vi "Unrock_Data_To_Cluster.vi"(0 "Test":sgl[][](array[numeric]), 1 "Dev":sgl[](array[numeric]), 2 "Inacc":sgl[](array[numeric]), 3 "DIN":string, 4 "HN":string[](array[string]), 5 "HS":sgl[](array[numeric]), 6 "TEMP":string, 7 "TV":sgl[][](array[numeric]), 8 "TSN":string, 9 "HV":sgl[](array[numeric]), 10 "MODE":string, 11 "REP":sgl[](array[numeric]), 13 "AVG":sgl[](array[numeric])) -> (14 "All_data_String":string[][](array[string]), 15 "输出簇":T1)   [LabVIEW 2019]
uses:
  Unrock_Cluster.ctl
  Test_load.ctl
  Hardness_test.ctl
  TEST.lvclass
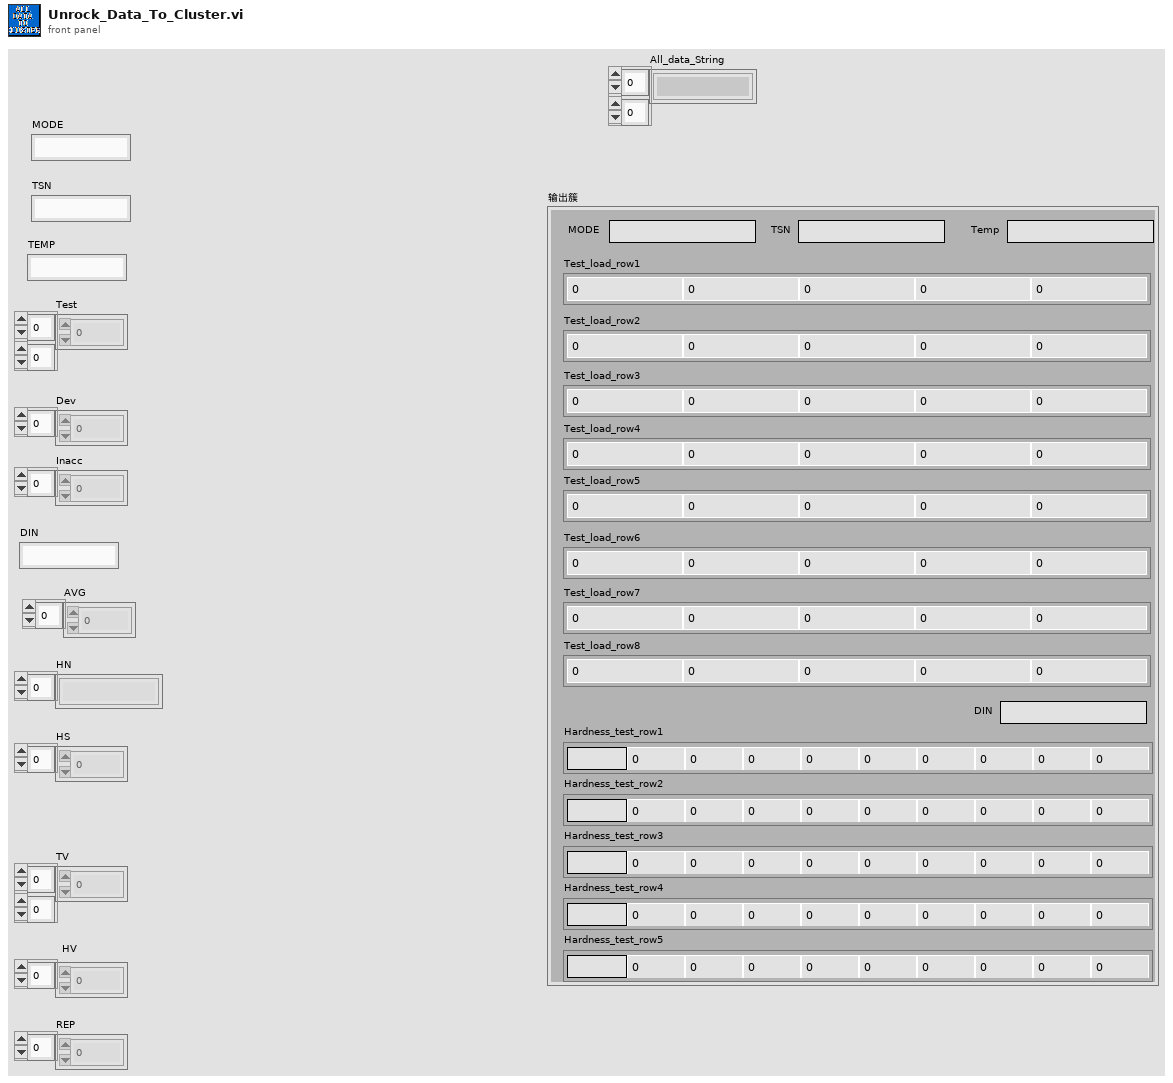
[diagram p1: front panel]
types:
  T1 = typedef "TEST.lvclass/Unrock_Cluster.ctl" = cluster{"MODE":string, "TSN":string, "Temp":string, "Test_load_row1":T2, "Test_load_row2":T2, "Test_load_row3":T2, "Test_load_row4":T2, "Test_load_row5":T2, "Test_load_row6":T2, "Test_load_row7":T2, "Test_load_row8":T2, "DIN":string, "Hardness_test_row1":T3, "Hardness_test_row2":T3, "Hardness_test_row3":T3, "Hardness_test_row4":T3, "Hardness_test_row5":T3}
  T2 = typedef "TEST.lvclass/Test_load.ctl" = cluster{"TEST1":sgl, "TEST2":sgl, "TEST3":sgl, "DEV":sgl, "INACC":sgl}
  T3 = typedef "TEST.lvclass/Hardness_test.ctl" = cluster{"HN":string, "HS":sgl, "TV1":sgl, "TV2":sgl, "TV3":sgl, "TV4":sgl, "TV5":sgl, "AVG":sgl, "HV":sgl, "REP":sgl}
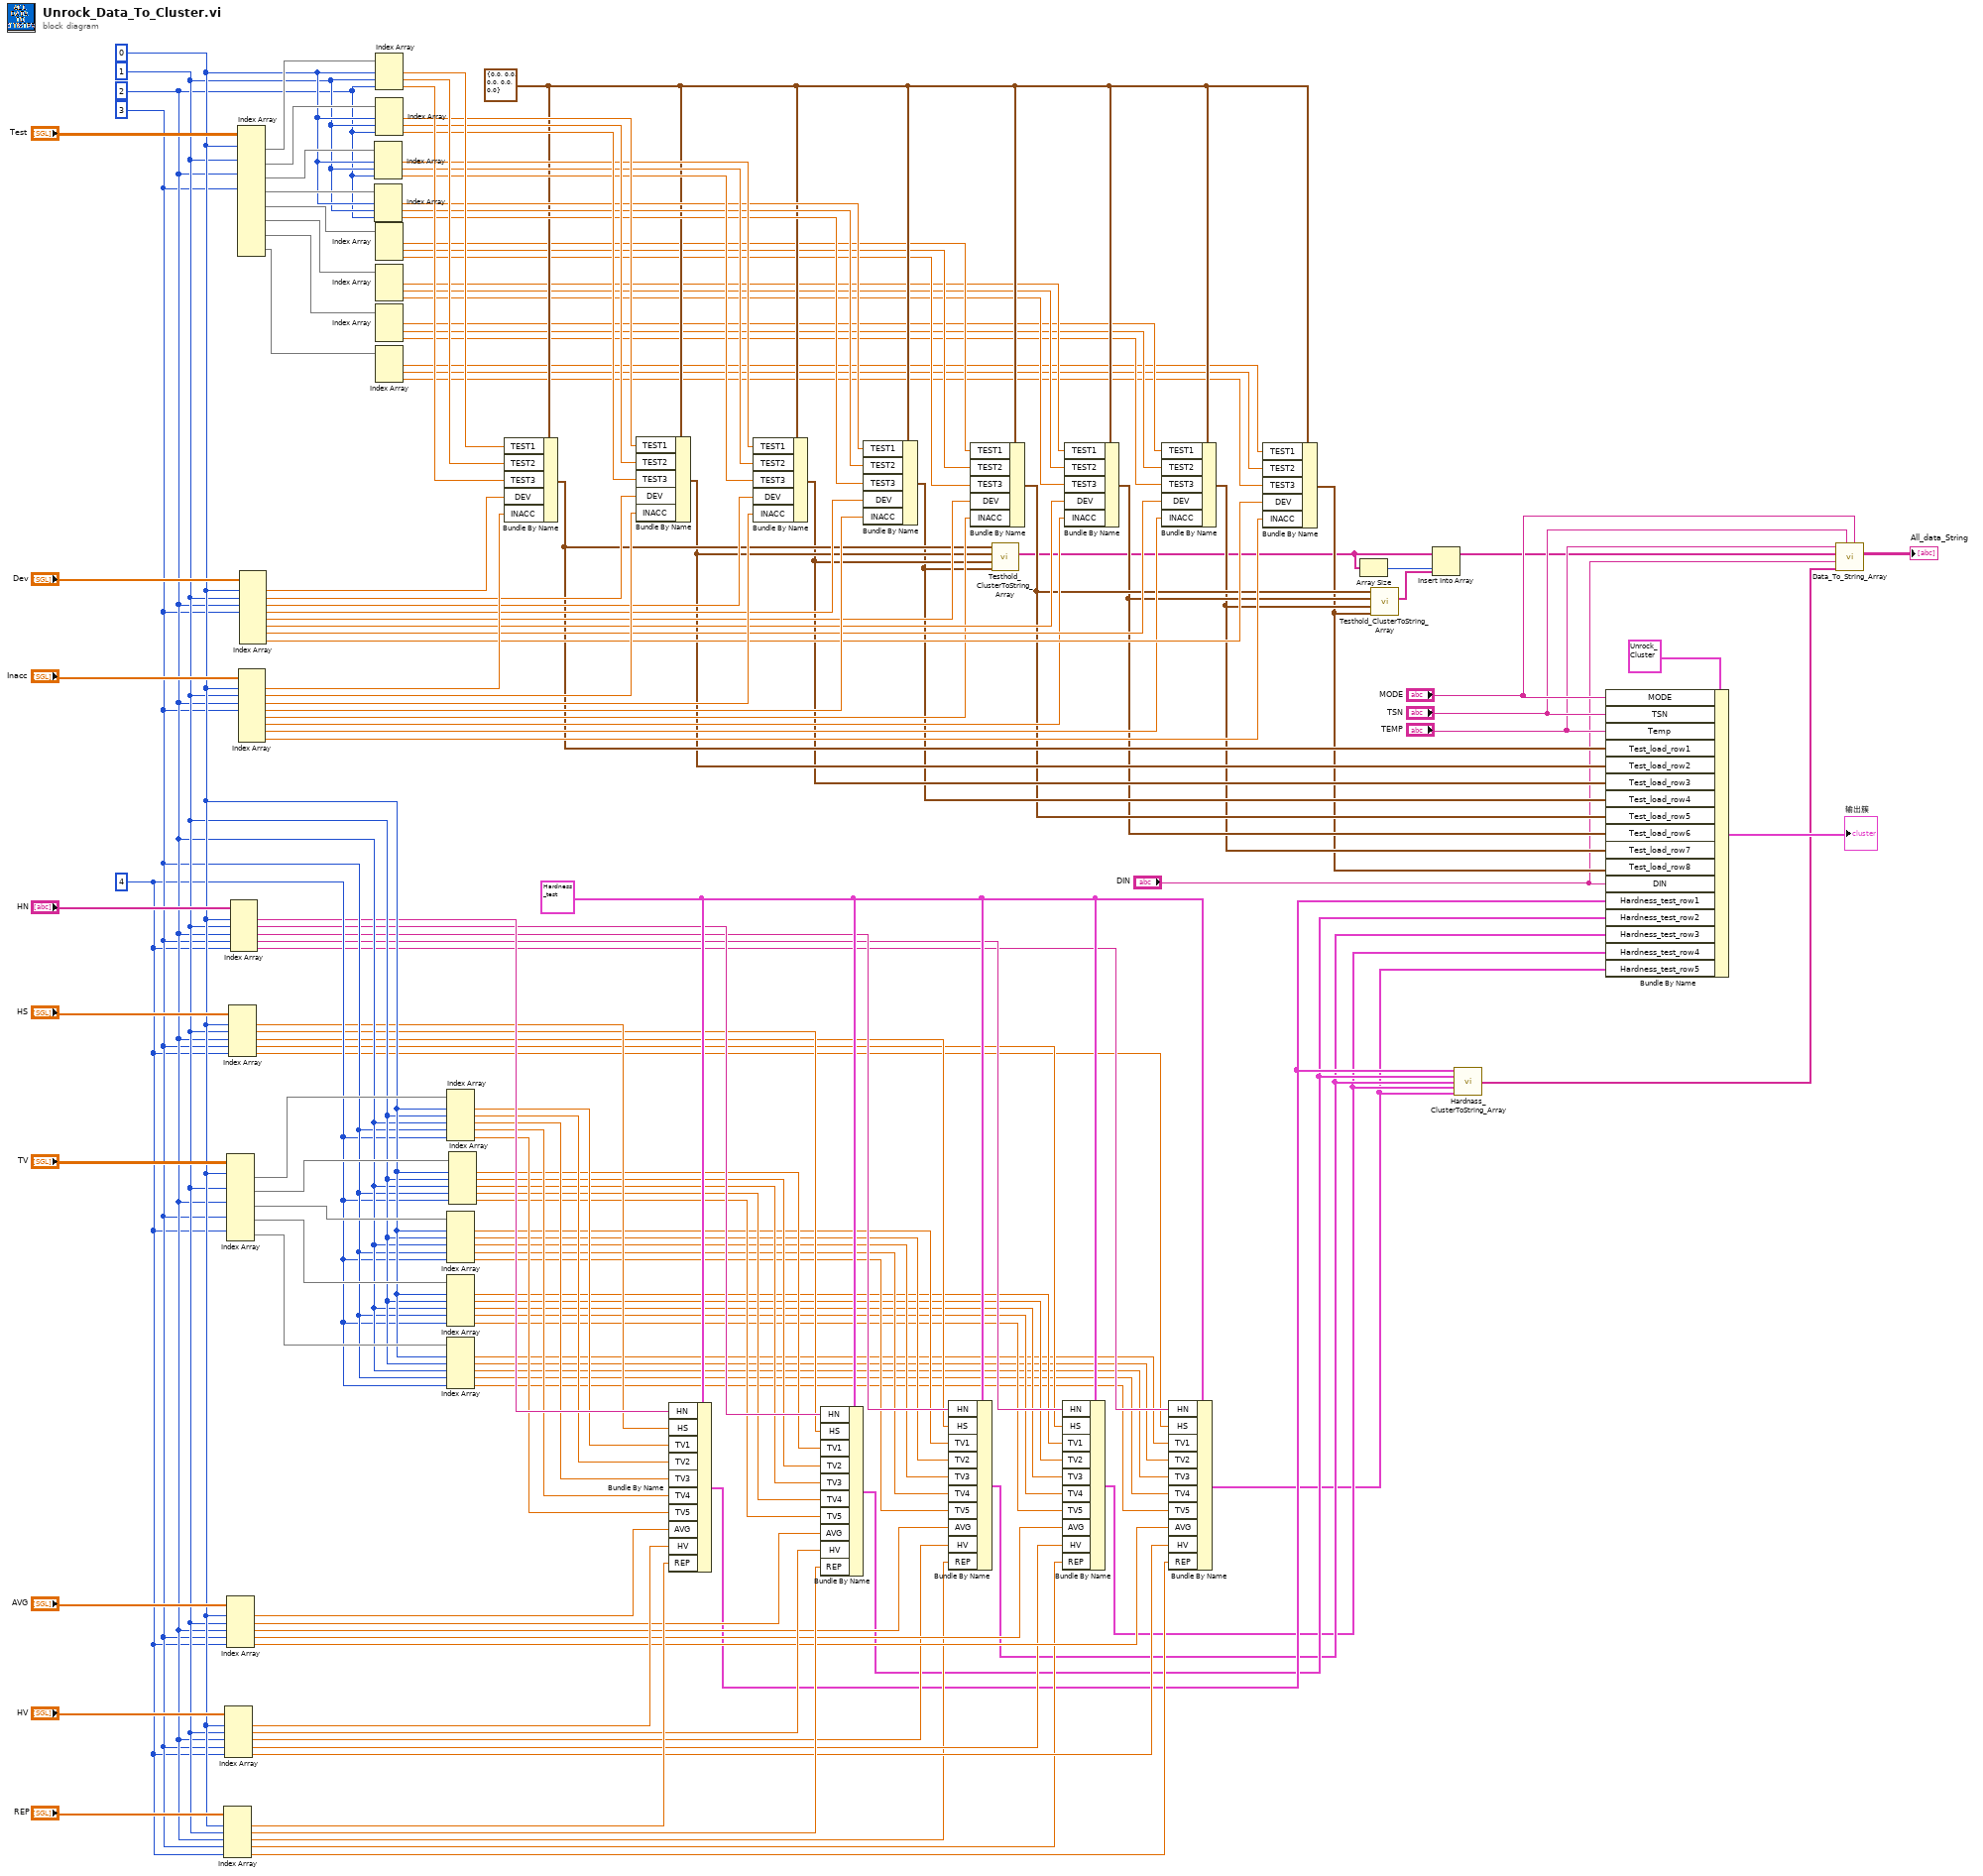
[diagram p0: block diagram]
diagram:
  w96 = T3 {"HN"="", "HS"=0.0, "TV1"=0.0, "TV2"=0.0, "TV3"=0.0, "TV4"=0.0, "TV5"=0.0, "AVG"=0.0, "HV"=0.0, "REP"=0.0} ("Hardness_test")
  w102 = 4
  w43 = T2 {"TEST1"=0.0, "TEST2"=0.0, "TEST3"=0.0, "DEV"=0.0, "INACC"=0.0} ("Test_load")
  w103 = 3 ("索引 (行)")
  w104 = 2 ("索引 (行)")
  w105 = 1 ("索引 (行)")
  w106 = 0 ("索引 (行)")
  n1 = Index Array(array="REP", index #1=w106, index #2=w105, index #3=w104, index #4=w103, index #5=w102) -> (element #1=w97:sgl, element #2=w91:sgl, element #3=w78:sgl, element #4=w77:sgl, element #5=w76:sgl)
  n2 = Index Array(array="HV", index #1=w106, index #2=w105, index #3=w104, index #4=w103, index #5=w102) -> (element #1=w98:sgl, element #2=w92:sgl, element #3=w81:sgl, element #4=w80:sgl, element #5=w79:sgl)
  n3 = Index Array(array="TV", index (row) #1=w106, index (row) #2=w105, index (row) #3=w104, index (row) #4=w103, index (row) #5=w102) -> (element #1=w111:sgl[], element #2=w110:sgl[], element #3=w109:sgl[], element #4=w108:sgl[], element #5=w107:sgl[])  [unwired: 5 in]
  n4 = Index Array(array="AVG", index #1=w106, index #2=w105, index #3=w104, index #4=w103, index #5=w102) -> (element #1=w99:sgl, element #2=w93:sgl, element #3=w84:sgl, element #4=w83:sgl, element #5=w82:sgl)
  n5 = Index Array(array="HS", index #1=w106, index #2=w105, index #3=w104, index #4=w103, index #5=w102) -> (element #1=w100:sgl, element #2=w94:sgl, element #3=w87:sgl, element #4=w86:sgl, element #5=w85:sgl)
  n6 = Index Array(array="HN", index #1=w106, index #2=w105, index #3=w104, index #4=w103, index #5=w102) -> (element #1=w101:string, element #2=w95:string, element #3=w90:string, element #4=w89:string, element #5=w88:string)
  n7 = Index Array(array="Test", index (row) #1=w106, index (row) #2=w105, index (row) #3=w104, index (row) #4=w103) -> (element #1=w141:sgl[], element #2=w140:sgl[], element #3=w139:sgl[], element #4=w138:sgl[], element #5=w42:sgl[], element #6=w41:sgl[], element #7=w40:sgl[], element #8=w39:sgl[])  [unwired: 12 in]
  n8 = Index Array(array="Inacc", index #1=w106, index #2=w105, index #3=w104, index #4=w103) -> (element #1=w133:sgl, element #2=w122:sgl, element #3=w120:sgl, element #4=w118:sgl, element #5=w22:sgl, element #6=w21:sgl, element #7=w20:sgl, element #8=w19:sgl)  [unwired: 4 in]
  n9 = Index Array(array="Dev", index #1=w106, index #2=w105, index #3=w104, index #4=w103) -> (element #1=w134:sgl, element #2=w123:sgl, element #3=w121:sgl, element #4=w119:sgl, element #5=w26:sgl, element #6=w25:sgl, element #7=w24:sgl, element #8=w23:sgl)  [unwired: 4 in]
  n10 = Index Array(array=w139, index #1=w106, index #2=w105, index #3=w104) -> (element #1=w129:sgl, element #2=w128:sgl, element #3=w127:sgl)
  n11 = Index Array(array=w138, index #1=w106, index #2=w105, index #3=w104) -> (element #1=w126:sgl, element #2=w125:sgl, element #3=w124:sgl)
  n12 = Index Array(array=w141, index #1=w106, index #2=w105, index #3=w104) -> (element #1=w137:sgl, element #2=w136:sgl, element #3=w135:sgl)
  n13 = Index Array(array=w140, index #1=w106, index #2=w105, index #3=w104) -> (element #1=w132:sgl, element #2=w131:sgl, element #3=w130:sgl)
  n14 = Index Array(array=w42) -> (element #1=w38:sgl, element #2=w37:sgl, element #3=w36:sgl)  [unwired: 3 in]
  n15 = Index Array(array=w41) -> (element #1=w35:sgl, element #2=w34:sgl, element #3=w33:sgl)  [unwired: 3 in]
  n16 = Index Array(array=w40) -> (element #1=w32:sgl, element #2=w31:sgl, element #3=w30:sgl)  [unwired: 3 in]
  n17 = Index Array(array=w39) -> (element #1=w29:sgl, element #2=w28:sgl, element #3=w27:sgl)  [unwired: 3 in]
  n18 = Index Array(array=w111, index #1=w106, index #2=w105, index #3=w104, index #4=w103, index #5=w102) -> (element #1=w70:sgl, element #2=w69:sgl, element #3=w68:sgl, element #4=w67:sgl, element #5=w66:sgl)
  n19 = Index Array(array=w109, index #1=w106, index #2=w105, index #3=w104, index #4=w103, index #5=w102) -> (element #1=w60:sgl, element #2=w59:sgl, element #3=w58:sgl, element #4=w57:sgl, element #5=w56:sgl)
  n20 = Index Array(array=w108, index #1=w106, index #2=w105, index #3=w104, index #4=w103, index #5=w102) -> (element #1=w55:sgl, element #2=w54:sgl, element #3=w53:sgl, element #4=w52:sgl, element #5=w51:sgl)
  n21 = Index Array(array=w107, index #1=w106, index #2=w105, index #3=w104, index #4=w103, index #5=w102) -> (element #1=w50:sgl, element #2=w49:sgl, element #3=w48:sgl, element #4=w47:sgl, element #5=w46:sgl)
  n22 = Index Array(array=w110, index #1=w106, index #2=w105, index #3=w104, index #4=w103, index #5=w102) -> (element #1=w65:sgl, element #2=w64:sgl, element #3=w63:sgl, element #4=w62:sgl, element #5=w61:sgl)
  n23 = Bundle By Name(cluster=w43, "TEST1"=w137, "TEST2"=w136, "TEST3"=w135, "DEV"=w134, "INACC"=w133) -> (w18:T2)
  n24 = Bundle By Name(cluster=w43, "TEST1"=w132, "TEST2"=w131, "TEST3"=w130, "DEV"=w123, "INACC"=w122) -> (w17:T2)
  n25 = Bundle By Name(cluster=w96, "HN"=w101, "HS"=w100, "TV1"=w70, "TV2"=w69, "TV3"=w68, "TV4"=w67, "TV5"=w66, "AVG"=w99, "HV"=w98, "REP"=w97) -> (w75:T3)
  n26 = Bundle By Name(cluster=w43, "TEST1"=w129, "TEST2"=w128, "TEST3"=w127, "DEV"=w121, "INACC"=w120) -> (w16:T2)
  n27 = Bundle By Name(cluster=w96, "HN"=w95, "HS"=w94, "TV1"=w65, "TV2"=w64, "TV3"=w63, "TV4"=w62, "TV5"=w61, "AVG"=w93, "HV"=w92, "REP"=w91) -> (w74:T3)
  n28 = Bundle By Name(cluster=w43, "TEST1"=w126, "TEST2"=w125, "TEST3"=w124, "DEV"=w119, "INACC"=w118) -> (w15:T2)
  n29 = Bundle By Name(cluster=w96, "HN"=w90, "HS"=w87, "TV1"=w60, "TV2"=w59, "TV3"=w58, "TV4"=w57, "TV5"=w56, "AVG"=w84, "HV"=w81, "REP"=w78) -> (w73:T3)
  n30 = Bundle By Name(cluster=w43, "TEST1"=w38, "TEST2"=w37, "TEST3"=w36, "DEV"=w26, "INACC"=w22) -> (w14:T2)
  n31 = call "Testhold_ClusterToString_Array.vi"("SLG_Cluster4"=w15, "SLG_Cluster3"=w16, "SLG_Cluster2"=w17, "SLG_Cluster"=w18) -> ("String_Array"=w9:string[])  [unwired: 7 in]
  n32 = Bundle By Name(cluster=w96, "HN"=w89, "HS"=w86, "TV1"=w55, "TV2"=w54, "TV3"=w53, "TV4"=w52, "TV5"=w51, "AVG"=w83, "HV"=w80, "REP"=w77) -> (w72:T3)
  n33 = Bundle By Name(cluster=w43, "TEST1"=w35, "TEST2"=w34, "TEST3"=w33, "DEV"=w25, "INACC"=w21) -> (w13:T2)
  n34 = Bundle By Name(cluster=w43, "TEST1"=w32, "TEST2"=w31, "TEST3"=w30, "DEV"=w24, "INACC"=w20) -> (w12:T2)
  n35 = Bundle By Name(cluster=w96, "HN"=w88, "HS"=w85, "TV1"=w50, "TV2"=w49, "TV3"=w48, "TV4"=w47, "TV5"=w46, "AVG"=w82, "HV"=w79, "REP"=w76) -> (w71:T3)
  n36 = Bundle By Name(cluster=w43, "TEST1"=w29, "TEST2"=w28, "TEST3"=w27, "DEV"=w23, "INACC"=w19) -> (w11:T2)
  n37 = Array Size(array=w9) -> (size(s)=w8:i32)
  n38 = call "Testhold_ClusterToString_Array.vi"("SLG_Cluster4"=w11, "SLG_Cluster3"=w12, "SLG_Cluster2"=w13, "SLG_Cluster"=w14) -> ("String_Array"=w10:string[])  [unwired: 7 in]
  n39 = Insert Into Array(array=w9, index=w8, new element=w10) -> (w4:string[])
  n40 = call "Hardnass_ClusterToString_Array.vi"("Hardness_test"=w75, "Hardness_test 2"=w74, "Hardness_test 3"=w73, "Hardness_test 4"=w72, "Hardness_test 5"=w71) -> ("StringArray"=w2:string[])  [unwired: 10 in]
  n41 = Bundle By Name(cluster=T1 {"MODE"="", "TSN"="", "Temp"="", "Test_load_row1"={"TEST1"=0.0, "TEST2"=0.0, "TEST3"=0.0, "DEV"=0.0, "INACC"=0.0}, "Test_load_row2"={"TEST1"=0.0, "TEST2"=0.0, "TEST3"=0.0, "DEV"=0.0, "INACC"=0.0}, "Test_load_row3"={"TEST1"=0.0, "TEST2"=0.0, "TEST3"=0.0, "DEV"=0.0, "INACC"=0.0}, "Test_load_row4"={"TEST1"=0.0, "TEST2"=0.0, "TEST3"=0.0, "DEV"=0.0, "INACC"=0.0}, "Test_load_row5"={"TEST1"=0.0, "TEST2"=0.0, "TEST3"=0.0, "DEV"=0.0, "INACC"=0.0}, "Test_load_row6"={"TEST1"=0.0, "TEST2"=0.0, "TEST3"=0.0, "DEV"=0.0, "INACC"=0.0}, "Test_load_row7"={"TEST1"=0.0, "TEST2"=0.0, "TEST3"=0.0, "DEV"=0.0, "INACC"=0.0}, "Test_load_row8"={"TEST1"=0.0, "TEST2"=0.0, "TEST3"=0.0, "DEV"=0.0, "INACC"=0.0}, "DIN"="", "Hardness_test_row1"={"HN"="", "HS"=0.0, "TV1"=0.0, "TV2"=0.0, "TV3"=0.0, "TV4"=0.0, "TV5"=0.0, "AVG"=0.0, "HV"=0.0, "REP"=0.0}, "Hardness_test_row2"={"HN"="", "HS"=0.0, "TV1"=0.0, "TV2"=0.0, "TV3"=0.0, "TV4"=0.0, "TV5"=0.0, "AVG"=0.0, "HV"=0.0, "REP"=0.0}, "Hardness_test_row3"={"HN"="", "HS"=0.0, "TV1"=0.0, "TV2"=0.0, "TV3"=0.0, "TV4"=0.0, "TV5"=0.0, "AVG"=0.0, "HV"=0.0, "REP"=0.0}, "Hardness_test_row4"={"HN"="", "HS"=0.0, "TV1"=0.0, "TV2"=0.0, "TV3"=0.0, "TV4"=0.0, "TV5"=0.0, "AVG"=0.0, "HV"=0.0, "REP"=0.0}, "Hardness_test_row5"={"HN"="", "HS"=0.0, "TV1"=0.0, "TV2"=0.0, "TV3"=0.0, "TV4"=0.0, "TV5"=0.0, "AVG"=0.0, "HV"=0.0, "REP"=0.0}} ("Unrock_Cluster"), "MODE"="MODE", "TSN"="TSN", "Temp"="TEMP", "Test_load_row1"=w18, "Test_load_row2"=w17, "Test_load_row3"=w16, "Test_load_row4"=w15, "Test_load_row5"=w14, "Test_load_row6"=w13, "Test_load_row7"=w12, "Test_load_row8"=w11, "DIN"="DIN", "Hardness_test_row1"=w75, "Hardness_test_row2"=w74, "Hardness_test_row3"=w73, "Hardness_test_row4"=w72, "Hardness_test_row5"=w71) -> (→"输出簇":T1)
  n42 = call "Data_To_String_Array.vi"("MODE"="MODE", "TSN"="TSN", "Hardness_string"=w2, "DIN"="DIN", "Test_load_string"=w4, "TEMP"="TEMP") -> ("String_Array"=→"All_data_String":string[][])  [unwired: 5 in]
